vi "Store Active Altitude Observer.vi"(8 "error in (no error)":errorcluster, 10 "Altitude Observer In":refnum<class "Observer.lvclass">, 11 "Vessel in":refnum<class "Vessel.lvclass">) -> (0 "error out":errorcluster, 3 "Vessel out":refnum<class "Vessel.lvclass">)   [LabVIEW 2014, in "Vessel.lvclass"]
uses:
  Vessel.lvclass
  Observer/Observer.lvclass
  Vessel.lvclass/Vessel.ctl
  Supervisor/Supervisor.lvclass
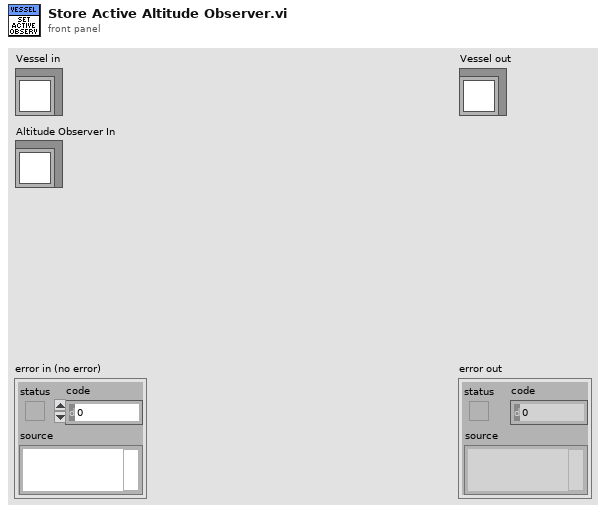
[diagram p1: front panel]
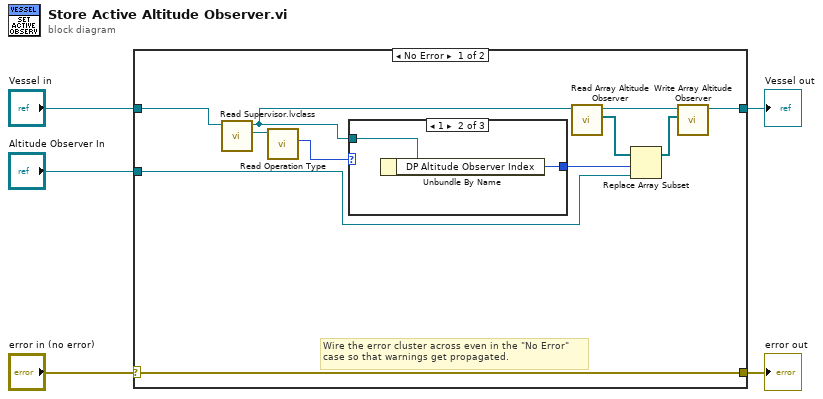
[diagram p0: block diagram]
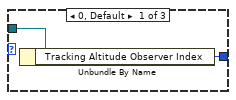
[diagram p2: hidden frame]
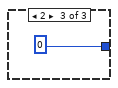
[diagram p3: hidden frame]
diagram:
  n1 = case shown="No Error" "error in (no error)" {
    selector: "error in (no error)" -> [w16 w23]
    tunnel: [w16 w23] -> w4
    tunnel: [w7 w22] -> w2
    tunnel: "Vessel in" -> [w15 w22]
    tunnel: "Altitude Observer In" -> [w12 _]
    frame No Error {
      # "Wire the error cluster across even in the \"No Error\"\ncase so that warnings get propagated."
      n2 = call "Read Supervisor.lvclass.vi"("Vessel in"=w15) -> ("Supervisor.lvclass"=w14:refnum<class "Supervisor.lvclass">, "Vessel out"=w9:refnum<class "Vessel.lvclass">)  [unwired: 8 in, 1 out]
      n3 = call-dynamic "Read Operation Type.vi"("Supervisor in"=w14) -> ("Operation Type"=w13:u16)  [unwired: 8 in, 2 out]
      n4 = case shown="1" w13 {
        tunnel: w9 -> [w18 w20 _]
        tunnel: [w17 w19 0] -> w11
        frame 0, Default {
          n5 = Unbundle By Name(w18) -> ("Tracking Altitude Observer Index"=w17:i32)
        }
        frame 1 {
          n6 = Unbundle By Name(w20) -> ("DP Altitude Observer Index"=w19:i32)
        }
        frame 2 {
        }
      }
      n7 = call-dynamic "Read Array Altitude Observer.vi"("Vessel in"=w9) -> ("Array Altitude Observer"=w10:refnum<class "Observer.lvclass">[], "Vessel out"=w6:refnum<class "Vessel.lvclass">)  [unwired: 8 in, 1 out]
      n8 = Replace Array Subset(array=w10, new element=w12, index=w11) -> (w8:refnum<class "Observer.lvclass">[])
      n9 = call-dynamic "Write Array Altitude Observer.vi"("Array Altitude Observer"=w8, "Vessel in"=w6) -> ("Vessel out"=w7:refnum<class "Vessel.lvclass">)  [unwired: 8 in, 1 out]
    }
    frame Error {
    }
  }
  "error out" <- w4
  "Vessel out" <- w2
